vi "T7_Read_Float_Registers.vi"(6 "Num Registers":u16=2, 8 "error in (no error)":errorcluster, 9 "FirstChannel":u16, 11 "IP Address(:port)":string="192.168.1.15") -> (0 "error out":errorcluster, 1 "ReadAt":timestamp, 2 "LastValue":dbl, 3 "Array":dbl[](array[numeric]))   [LabVIEW 2018]
uses:
  <vilib>/Plasmionique/MB Master/MB_Master_TCP/MB_Master_TCP.lvclass
  Applications/National Instruments/LabVIEW 2018 64-bit/vi.lib/Plasmionique/MB Master/MB_Master/MB_Master.lvclass
  <vilib>/Plasmionique/MB Master/MB Master.lvlib
panel:
  out "Starting Address":u16
  out "Results (binary)":u16[](array[numeric])
  # "Slave Read-only Registers"
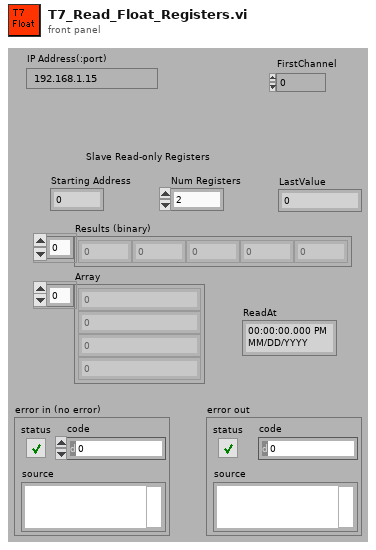
[diagram p1: front panel]
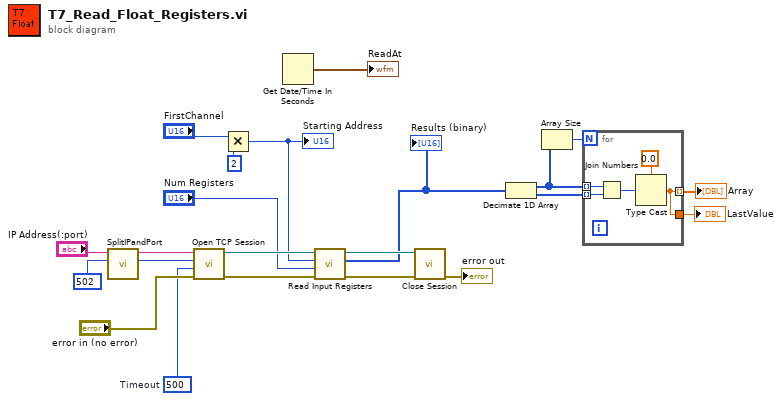
[diagram p0: block diagram]
diagram:
  w12 = 500  # Timeout
  n1 = call "SplitIPandPort.vi"("defaultPort(10001)"=u16 502, "IP:Port"="IP Address(:port)") -> ("Port"=w8:u16, "IP"=w9:string)  [unwired: 8 in]
  n2 = call <vilib>:"Open TCP Session.vi"("error in (no error)"="error in (no error)", "Timeout (10000)"=w12, "Port (502)"=w8, "IP Address"=w9) -> ("error out"=w21:errorcluster, "MB_TCP session"=w22:refnum<class "MB_Master_TCP.lvclass">)  [unwired: 6 in]
  n3 = Multiply(x="FirstChannel", y=u16 2) -> (x*y=w13:u16)
  "Starting Address" <- w13
  n4 = Get Date/Time In Seconds() -> (seconds since 1Jan1904=→"ReadAt":timestamp)
  n5 = call <vilib>:"Read Input Registers.vi"("error in (no error)"=w21, "quantity"="Num Registers", "starting address"=w13, "MB session in"=w22) -> ("error out"=w20:errorcluster, "Registers"=w1:u16[], "MB session out"=w19:refnum<class "MB_Master_TCP.lvclass">)  [unwired: 5 in]
  "Results (binary)" <- w1
  n6 = call-dynamic "Close Session.vi"("error in (no error)"=w20, "MB TCP session"=w19) -> ("error out"=→"error out":errorcluster)  [unwired: 9 in]
  n7 = Decimate 1D Array(w1) -> (w6:u16[], w5:u16[])
  n8 = Array Size(array=w6) -> (size(s)=w7:i32)
  n9 = for {
    N: w7 -> [_]
    tunnel: w6 -> [w26] mode=indexing
    tunnel: w5 -> [w27] mode=indexing
    tunnel: [w23] -> w4 mode=indexing
    tunnel: [w23] -> w3
    n10 = Join Numbers(hi=w26, lo=w27) -> ((hi.lo)=w25:u32)
    n11 = Type Cast(type=sgl 0.0, x=w25) -> (*(type *) &x=w23:sgl)
  }
  "Array" <- w4
  "LastValue" <- w3
